vi "Three-Phase Measurement System.vi"() -> ()   [LabVIEW 2020]
uses:
  <vilib>/MakerHub/LINX/Public/Peripherals/Analog/Analog Read N Chans.vi
  <vilib>/MakerHub/LINX/Private/Local IO/LinxAnalogRead.vi
  <vilib>/MakerHub/LINX/Public/Utilities/Check Channel.vi
  <vilib>/MakerHub/LINX/Public/Utilities/Open Serial.vi
  <vilib>/MakerHub/LINX/Private/Utilties/Generate Error.vi
  <vilib>/MakerHub/LINX/LMH-LINX.lvlib
panel:
  in  "?":T1(tab)
  out "Ph 3":dbl(knob) scale=-25.0..25.0
  out "i3":dbl(knob) scale=0.0..16.0
  out "Ph 2":dbl(knob) scale=-25.0..25.0
  out "i2":dbl(knob) scale=0.0..16.0
  out "Ph 1":dbl(knob) scale=-25.0..25.0
  out "i1":dbl(knob) scale=0.0..16.0
  out "vector diagram":cluster{dbl[], dbl[]}[](graph) caption="THREE-PHASE SYSTEMS \n\n\n\n\nThree Phase Measurement System"
  in  "Serial Port":refnum<visa-resource-name>="N/A"
  in  "AI Channel":u8[](array[numeric])
  in  "?":bool
  in  "START":bool
  out "OSCILLOSCOPE":dynamicdata(graph)
  out "i1 2":dbl(knob) scale=0.0..16.0
  out "Ph 1":dbl(knob) scale=-25.0..25.0
  out "i2":dbl(knob) scale=0.0..16.0
  out "Ph 2":dbl(knob) scale=-25.0..25.0
  out "i3 2":dbl(knob) scale=0.0..16.0
  out "Ph 3":dbl(knob) scale=-25.0..25.0
  in  "?":bool
  out "Analog Data 2":T2(graph)
  in  "?":bool
  out "i1/A A":dbl
  out "i2/A":dbl
  out "i3/A":dbl
  out "Ph i1°":dbl
  out "Ph i2°":dbl
  out "Ph i3°":dbl
  out "u1/V":dbl
  out "u2/V":dbl
  out "u3/V":dbl
  out "i1 m /A":dbl
  out "i2 m /A":dbl
  out "i3 m /A":dbl
  out "ph u2°":dbl
  out "ph u3°":dbl
  out "ph i1m°":dbl
  out "ph i2m°":dbl
  out "ph i3m°":dbl
  out "ph u1°":dbl
  out "Ph 3":dbl(knob) scale=-25.0..25.0
  out "i3 3":dbl(knob) scale=0.0..16.0
  out "Ph 2":dbl(knob) scale=-25.0..25.0
  out "i2":dbl(knob) scale=0.0..16.0
  out "Ph 1":dbl(knob) scale=-25.0..25.0
  out "i1 3":dbl(knob) scale=0.0..16.0
  in  "?":bool
  # "INPUT DATA SIMULATION"
  # "NUMERICAL DATA"
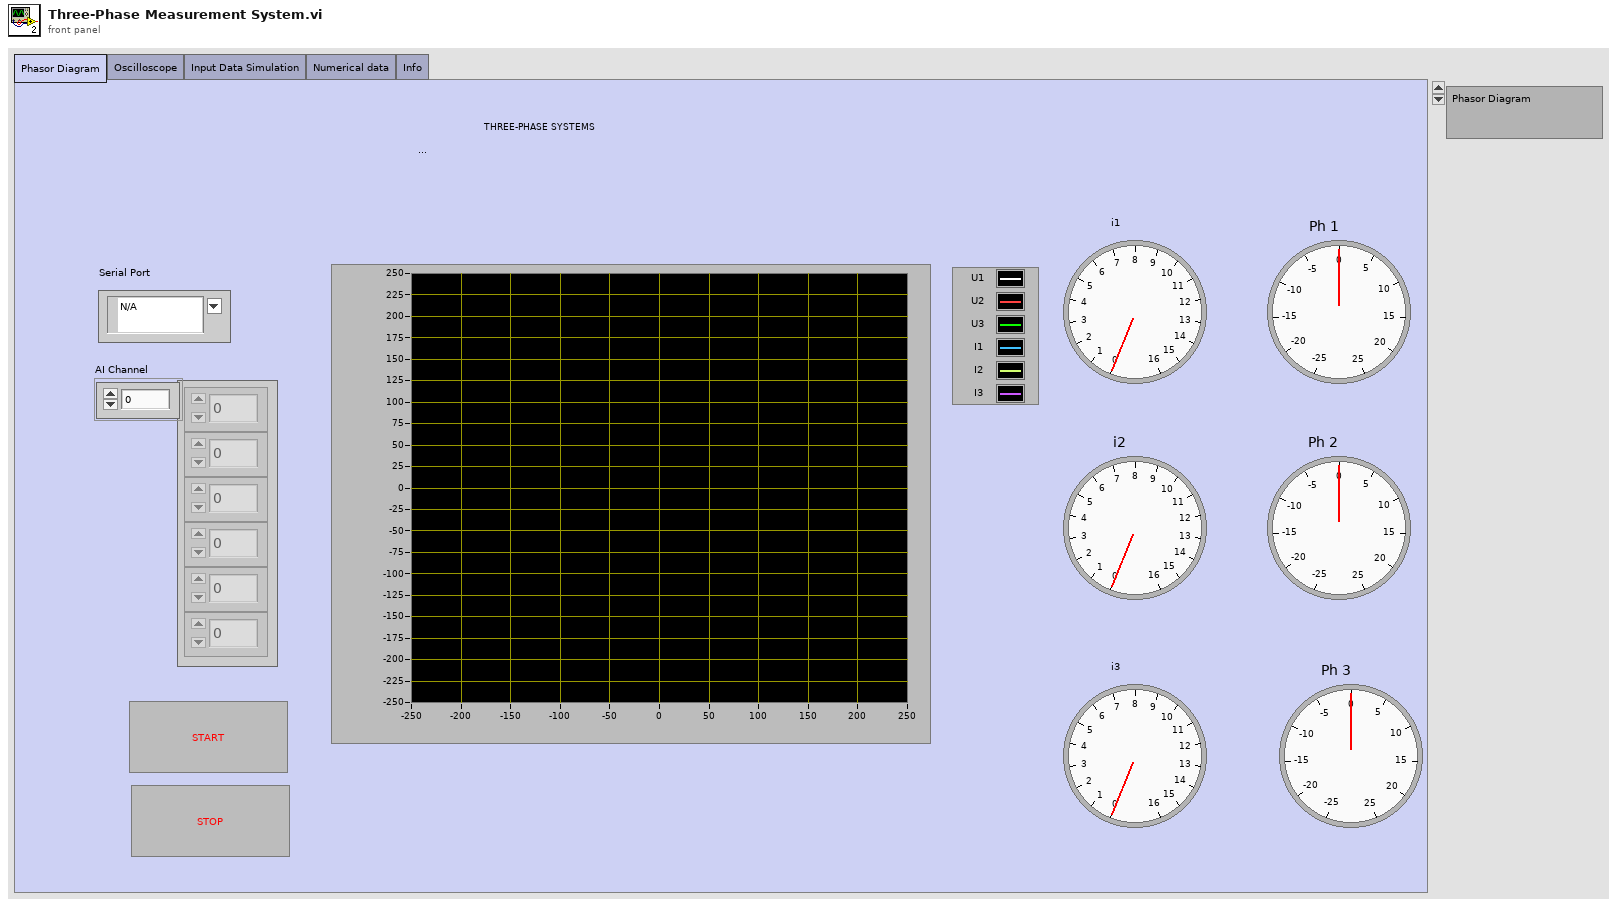
[diagram p1: front panel]
types:
  T1 = enum32{"Phasor Diagram", "Oscilloscope", "Input Data Simulation", "Numerical data", "Info"}
  T2 = cluster{"Voltages[0]":dbl, "Voltages[1]":dbl, "Voltages[2]":dbl, "Voltages[3]":dbl, "Voltages[4]":dbl, "Voltages[5]":dbl, "Voltages[6]":dbl, "Voltages[7]":dbl, "Voltages[8]":dbl}
  T3 = typedef "LMH-LINX.lvlib/LINX Ref.ctl" = cluster{"IO":T4, "Interface":T5, "LINX Device Config":T6}
  T4 = typedef "LMH-LINX.lvlib/Platform.ctl" = enum16{"Remote", "Local"}
  T5 = typedef "LMH-LINX.lvlib/Interface.ctl" = enum16{"Serial", "TCP"}
  T6 = typedef "LMH-LINX.lvlib/Device.lvlib/LINX Device Config.ctl" = cluster{"Interface":T5, "COM Port":refnum<visa-resource-name>, "TCP Configuration":T7, "Device Family":u8, "Device ID":u8, "Device Name":string, "TCP Ref":refnum<k5>, "Channels":T8}
  T7 = typedef "LMH-LINX.lvlib/Device.lvlib/TCP Config.ctl" = cluster{"IP Address":string, "Port":u16}
  T8 = typedef "LMH-LINX.lvlib/Channels.ctl" = cluster{"DI":u8[], "DO":u8[], "AI":u8[], "AO":u8[], "PWM":u8[], "QE":u8[], "UART":u8[], "I2C 2":u8[], "SPI":u8[], "CAN":u8[], "Servo":u8[], "AI Ref (V)":dbl, "AI Resolution (Bits)":u8, "AO Ref (V)":dbl, "AO Resolution (Bits)":u8}
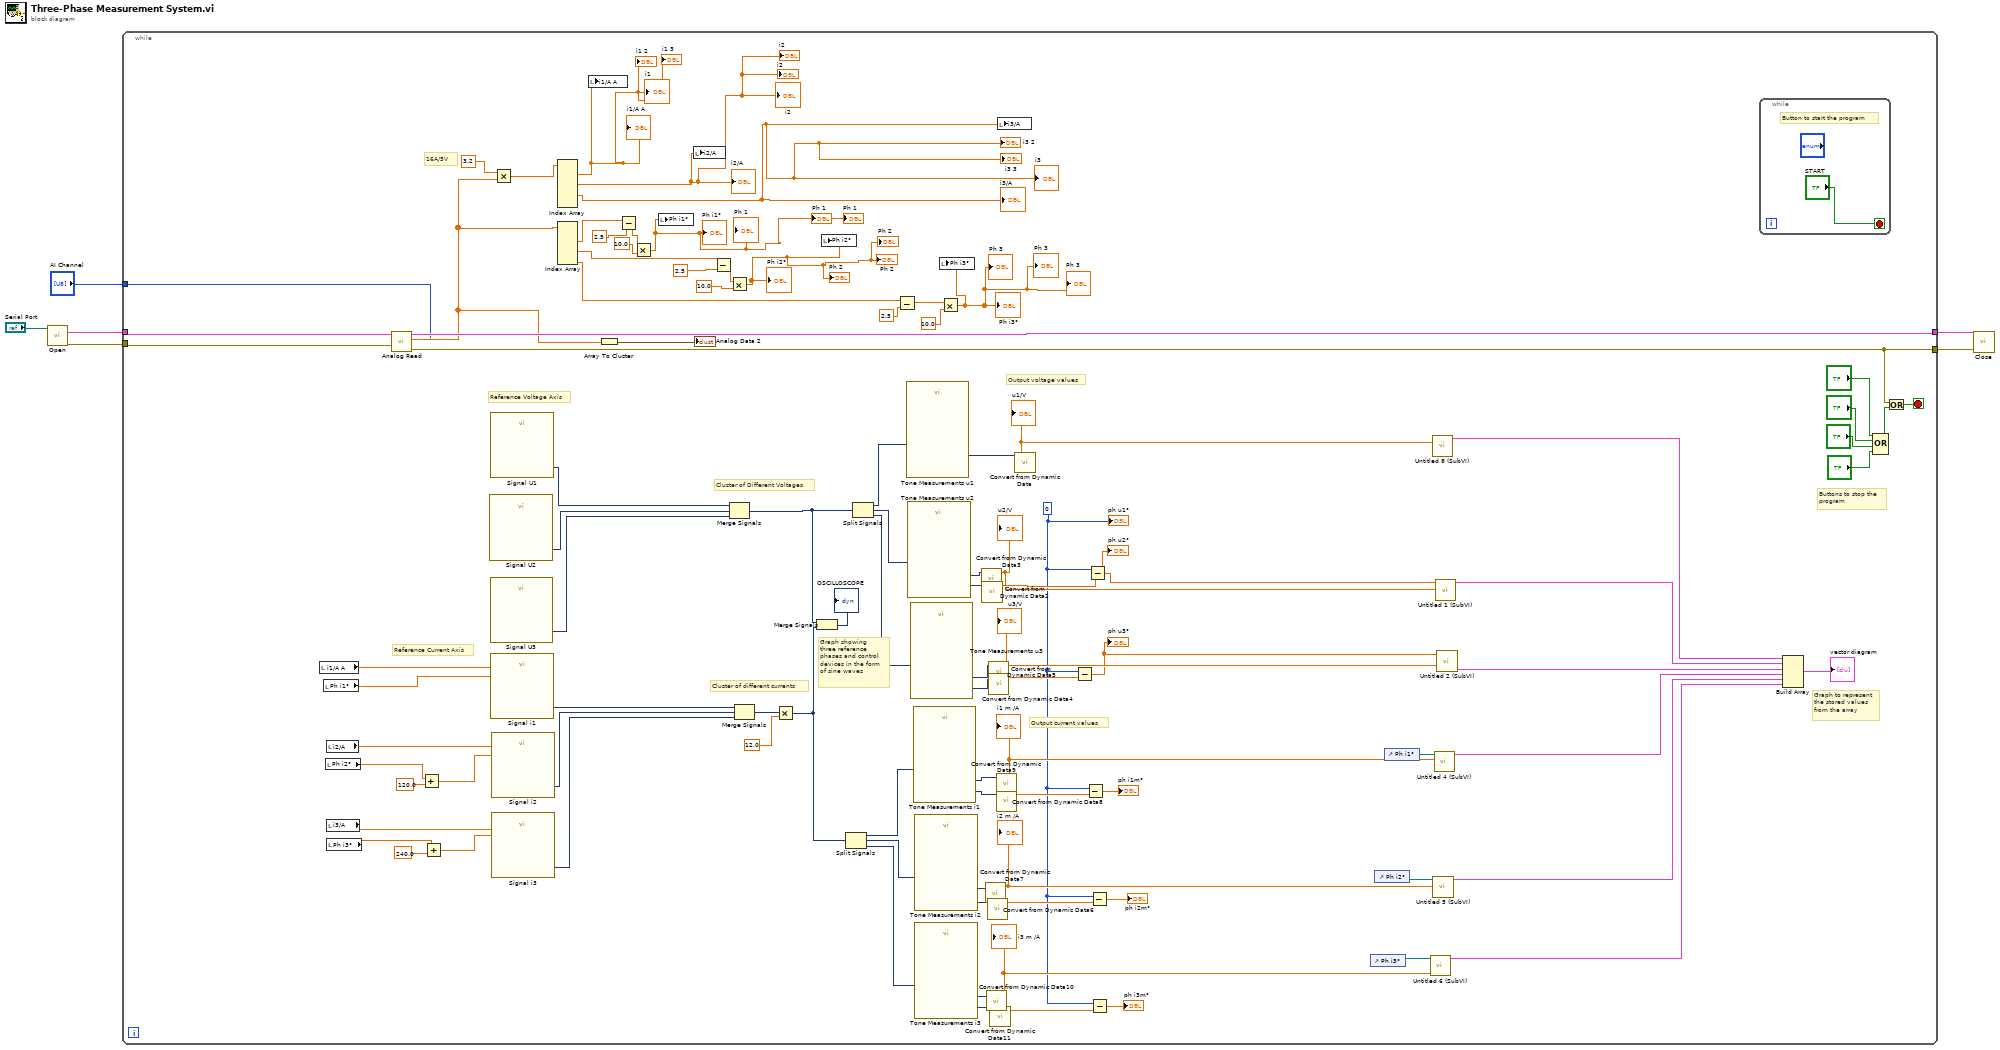
[diagram p0: block diagram]
diagram:
  n1 = call-poly <vilib>:"Open.vi"("Serial Port"="Serial Port") -> ("Error Out"=w4:errorcluster, "LINX Resource"=w5:T3)  [unwired: 8 in, 1 out]
  n2 = while {
    tunnel: w5 -> [w104]
    tunnel: w4 -> [w103]
    tunnel: [w83] -> w3
    tunnel: "AI Channel" -> [w64]
    tunnel: [w24] -> w1
    stop <- w23 stop-if-true
    w30 = 0
    # "Buttons to stop the\nprogram"
    # "Graph to represent\nthe stored values\nfrom the array"
    # "Output current values"
    # "Output voltage values"
    # "Graph showing\nthree reference \nphases and control \ndevices in the form \nof sine waves"
    # "Cluster of different currents"
    # "Cluster of Different Voltages"
    # "Reference Current Axis"
    # "Reference Voltage Axis"
    # "16A/5V"
    n3 = local read "i1/A A"() -> (w89:dbl)
    n4 = local read "Ph i1°"() -> (w88:dbl)
    n5 = local read "Ph i2°"() -> (w80:dbl)
    n6 = local read "i2/A"() -> (w87:dbl)
    n7 = local read "i3/A"() -> (w86:dbl)
    n8 = local read "Ph i3°"() -> (w82:dbl)
    n9 = call-poly <vilib>:"Analog Read.vi"("Error In"=w103, "AI Channel(s)"=w64, "LINX Resource"=w104) -> ("Error Out"=w24:errorcluster, "Voltages"=w68:dbl[], "LINX Resource"=w83:T3)  [unwired: 5 in, 1 out]
    n10 = Add(x=w80, y=120.0) -> (x+y=w78:dbl)
    n11 = Add(x=w82, y=240.0) -> (x+y=w81:dbl)
    n12 = call "Signal U2"() -> ("Sine"=w91:dynamicdata)  [unwired: 14 in, 1 out]
    n13 = call "Signal U3"() -> ("Sine"=w90:dynamicdata)  [unwired: 14 in, 1 out]
    n14 = call "Signal U1"() -> ("Sine"=w92:dynamicdata)  [unwired: 14 in, 1 out]
    n15 = call "Signal i1"("Amplitude"=w89, "Phase"=w88) -> ("Sine"=w67:dynamicdata)  [unwired: 12 in, 1 out]
    n16 = call "Signal i2"("Amplitude"=w87, "Phase"=w78) -> ("Sine"=w66:dynamicdata)  [unwired: 12 in, 1 out]
    n17 = call "Signal i3"("Amplitude"=w86, "Phase"=w81) -> ("Sine"=w65:dynamicdata)  [unwired: 12 in, 1 out]
    n18 = Multiply(x=3.2, y=w68) -> (x*y=w101:dbl[])
    n19 = Index Array(array=w101) -> (element #1=w20:dbl, element #3=w19:dbl, element #5=w18:dbl)  [unwired: 7 in, 4 out]
    "i1/A A" <- w20
    "i2/A" <- w19
    "i3/A" <- w18
    "i1" <- w20
    "i2" <- w19
    "i3" <- w18
    "i1 2" <- w20
    "i2" <- w19
    "i3 2" <- w18
    "i3 3" <- w18
    "i2" <- w19
    "i1 3" <- w20
    n20 = Index Array(array=w68) -> (element #2=w99:dbl, element #4=w32:dbl, element #6=w31:dbl)  [unwired: 6 in, 3 out]
    n21 = local write "i1/A A"(w20) -> ()
    n22 = Array To Cluster(array=w68) -> (cluster=→"Analog Data 2":T2)
    n23 = Subtract(x=w99, y=2.5) -> (x-y=w100:dbl)
    n24 = Multiply(x=w100, y=10.0) -> (x*y=w21:dbl)
    "Ph i1°" <- w21
    "Ph 1" <- w21
    "Ph 1" <- w21
    "Ph 1" <- w21
    n25 = local write "Ph i1°"(w21) -> ()
    n26 = local write "i2/A"(w19) -> ()
    n27 = Subtract(x=w32, y=2.5) -> (x-y=w96:dbl)
    n28 = Multiply(x=w96, y=10.0) -> (x*y=w12:dbl)
    "Ph i2°" <- w12
    "Ph 2" <- w12
    "Ph 2" <- w12
    "Ph 2" <- w12
    n29 = Merge Signals(w92, w91, w90) -> (w84:dynamicdata)
    n30 = Merge Signals(w67, w66, w65) -> (w77:dynamicdata)
    n31 = Multiply(x=w77, y=12.0) -> (x*y=w25:dynamicdata)
    n32 = Merge Signals(w84, w25) -> (→"OSCILLOSCOPE":dynamicdata)
    n33 = local write "Ph i2°"(w12) -> ()
    n34 = Split Signals(w25) -> (w35:dynamicdata, w34:dynamicdata, w33:dynamicdata)  [unwired: 3 in]
    n35 = Split Signals(w84) -> (w76:dynamicdata, w75:dynamicdata, w74:dynamicdata)  [unwired: 3 in]
    n36 = Subtract(x=w31, y=2.5) -> (x-y=w93:dbl)
    n37 = call "Tone Measurements u1"("Signals"=w76) -> ("Amplitude"=w73:dynamicdata)  [unwired: 8 in, 2 out]
    n38 = call "Tone Measurements u2"("Signals"=w75) -> ("Phase"=w69:dynamicdata, "Amplitude"=w70:dynamicdata)  [unwired: 8 in, 1 out]
    n39 = call "Tone Measurements u3"("Signals"=w74) -> ("Phase"=w71:dynamicdata, "Amplitude"=w72:dynamicdata)  [unwired: 8 in, 1 out]
    n40 = call "Tone Measurements i1"("Signals"=w35) -> ("Phase"=w59:dynamicdata, "Amplitude"=w58:dynamicdata)  [unwired: 8 in, 1 out]
    n41 = call "Tone Measurements i2"("Signals"=w34) -> ("Phase"=w60:dynamicdata, "Amplitude"=w61:dynamicdata)  [unwired: 8 in, 1 out]
    n42 = call "Tone Measurements i3"("Signals"=w33) -> ("Phase"=w63:dynamicdata, "Amplitude"=w62:dynamicdata)  [unwired: 8 in, 1 out]
    n43 = Multiply(x=w93, y=10.0) -> (x*y=w22:dbl)
    "Ph i3°" <- w22
    "Ph 3" <- w22
    "Ph 3" <- w22
    "Ph 3" <- w22
    n44 = local write "Ph i3°"(w22) -> ()
    n45 = call "Convert from Dynamic Data3"("Dynamic Data Type"=w70) -> ("Scalar"=w50:dbl)  [unwired: 3 in]
    "u2/V" <- w50
    n46 = call "Convert from Dynamic Data2"("Dynamic Data Type"=w69) -> ("Scalar"=w57:dbl)  [unwired: 3 in]
    n47 = call "Convert from Dynamic Data7"("Dynamic Data Type"=w61) -> ("Scalar"=w46:dbl)  [unwired: 3 in]
    "i2 m /A" <- w46
    n48 = call "Convert from Dynamic Data10"("Dynamic Data Type"=w62) -> ("Scalar"=w45:dbl)  [unwired: 3 in]
    "i3 m /A" <- w45
    n49 = call "Convert from Dynamic Data6"("Dynamic Data Type"=w60) -> ("Scalar"=w54:dbl)  [unwired: 3 in]
    n50 = call "Convert from Dynamic Data5"("Dynamic Data Type"=w72) -> ("Scalar"=w49:dbl)  [unwired: 3 in]
    "u3/V" <- w49
    n51 = call "Convert from Dynamic Data4"("Dynamic Data Type"=w71) -> ("Scalar"=w56:dbl)  [unwired: 3 in]
    n52 = call "Convert from Dynamic Data11"("Dynamic Data Type"=w63) -> ("Scalar"=w53:dbl)  [unwired: 3 in]
    n53 = call "Convert from Dynamic Data9"("Dynamic Data Type"=w58) -> ("Scalar"=w38:dbl)  [unwired: 3 in]
    "i1 m /A" <- w38
    n54 = call "Convert from Dynamic Data8"("Dynamic Data Type"=w59) -> ("Scalar"=w55:dbl)  [unwired: 3 in]
    n55 = local write "i3/A"(w18) -> ()
    n56 = call "Convert from Dynamic Data"("Dynamic Data Type"=w73) -> ("Scalar"=w14:dbl)  [unwired: 3 in]
    "u1/V" <- w14
    n57 = Subtract(x=w30, y=w56) -> (x-y=w48:dbl)
    "ph u3°" <- w48
    n58 = Subtract(x=w30, y=w55) -> (x-y=→"ph i1m°":dbl)
    n59 = Subtract(x=w30, y=w57) -> (x-y=w51:dbl)
    "ph u2°" <- w51
    n60 = Subtract(x=w30, y=w54) -> (x-y=→"ph i2m°":dbl)
    n61 = Subtract(x=w30, y=w53) -> (x-y=→"ph i3m°":dbl)
    n62 = control-ref of="Ph i3°"() -> (w15:refnum<vi>)
    n63 = control-ref of="Ph i2°"() -> (w16:refnum<vi>)
    n64 = control-ref of="Ph i1°"() -> (w17:refnum<vi>)
    n65 = call "Untitled 6 (SubVI).vi"("Scalar"=w45, "Digital in"=w15) -> ("Cluster"=w39:cluster{dbl[], dbl[]})  [unwired: 9 in]
    n66 = call "Untitled 8 (SubVI).vi"("Scalar"=w14) -> ("Cluster"=w44:cluster{dbl[], dbl[]})  [unwired: 10 in]
    n67 = call "Untitled 5 (SubVI).vi"("Scalar"=w46, "Digital in"=w16) -> ("Cluster"=w40:cluster{dbl[], dbl[]})  [unwired: 9 in]
    n68 = call "Untitled 4 (SubVI).vi"("Scalar"=w38, "Digital in"=w17) -> ("Cluster"=w41:cluster{dbl[], dbl[]})  [unwired: 9 in]
    n69 = call "Untitled 1 (SubVI).vi"("Scalar"=w50, "Numeric"=w51) -> ("Cluster"=w43:cluster{dbl[], dbl[]})  [unwired: 9 in]
    n70 = call "Untitled 2 (SubVI).vi"("Scalar"=w49, "Numeric"=w48) -> ("Cluster"=w42:cluster{dbl[], dbl[]})  [unwired: 9 in]
    n71 = while {
      stop <- "START" stop-if-true
      # "Button to start the program"
    }
    n72 = Build Array "Build Array"(w44, w43, w42, w41, w40, w39) -> (→"vector diagram":cluster{dbl[], dbl[]}[])
    n73 = Compound Arithmetic op=OR("?", "?", "?", "?") -> (w7:bool)
    n74 = Or(x=w24, y=w7) -> (x .or. y?=w23:bool)
    "ph u1°" <- w30
  }
  n75 = call <vilib>:"Close.vi"("Error In"=w1, "LINX Resource"=w3) -> ()  [unwired: 9 in, 1 out]
